vi "GetHelp.vi"(11 "Solution Builder Operation in":refnum<class "Solution Builder Operation.lvclass">) -> (2 "Help":string, 3 "Solution Builder Operation out":refnum<class "Solution Builder Operation.lvclass">)   [LabVIEW 2019, in "Solution Builder Operation.lvclass"]
uses:
  Solution Builder Operation.lvclass
  <nishared>/LabVIEW CLI/Operations/CoreOperation/CoreOperation.lvclass
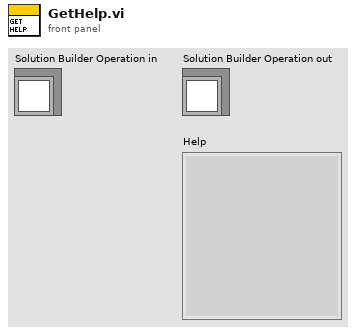
[diagram p1: front panel]
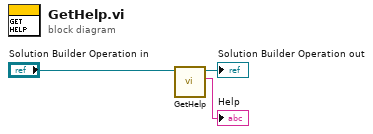
[diagram p0: block diagram]
diagram:
  n1 = call-parent "GetHelp.vi"("CoreOperation in"="Solution Builder Operation in") -> ("Help"=→"Help":string, "CoreOperation out"=→"Solution Builder Operation out":refnum<class "Solution Builder Operation.lvclass">)  [unwired: 9 in]
